vi "Get Ctrl Index.vi"(10 "Label":string, 11 "Panel Actor Template in":refnum<class "Network Management UI.lvclass">) -> (2 "Index":i32, 3 "Panel Actor Template out":refnum<class "Network Management UI.lvclass">)   [LabVIEW 2020, in "Network Management UI.lvlib" / "Network Management UI.lvclass"]
uses:
  Network Management UI.lvclass
  Network Management UI.lvclass/Network Management UI.ctl
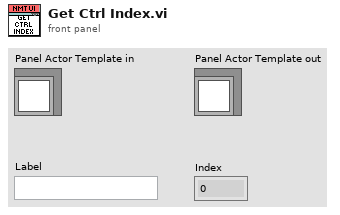
[diagram p1: front panel]
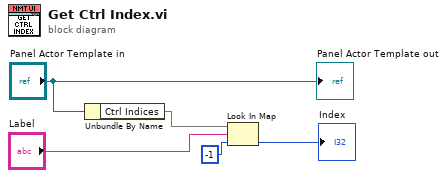
[diagram p0: block diagram]
diagram:
  n1 = Unbundle By Name("Panel Actor Template in") -> ("Ctrl Indices"=w4:map{string, i32})
  n2 = Look In Map(map=w4, key="Label", default value=-1) -> (value=→"Index":i32)  [unwired: 1 out]
  "Panel Actor Template out" <- "Panel Actor Template in"
